vi "Write Setpoint Temperature.vi"(8 "error in (no error)":errorcluster, 9 "Update Time":timestamp, 10 "Setpoint Temperature [degC]":dbl, 11 "Thermal Chamber Response Simlator In":refnum<class "Thermal Chamber Response Simlator.lvclass">) -> (0 "error out":errorcluster, 3 "Thermal Chamber Response Simlator Out":refnum<class "Thermal Chamber Response Simlator.lvclass">)   [LabVIEW 2020, in "Thermal Chamber Response Simlator.lvclass"]
uses:
  Thermal Chamber Response Simlator.lvclass
  Thermal Chamber Response Simlator.lvclass/Thermal Chamber Response Simlator.ctl
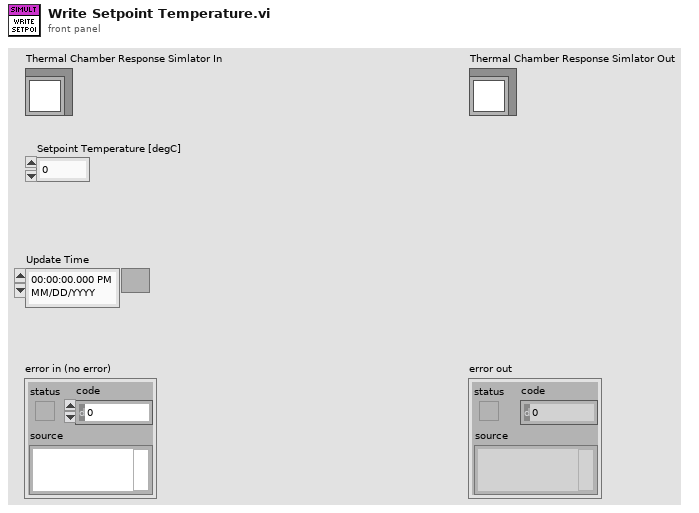
[diagram p1: front panel]
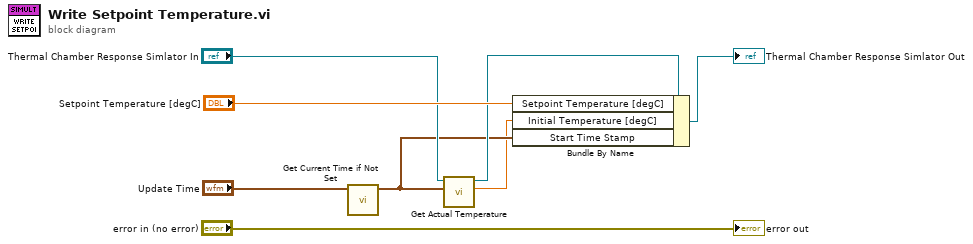
[diagram p0: block diagram]
diagram:
  n1 = call "Get Current Time if Not Set.vi"("Start Time"="Update Time") -> ("seconds since 1Jan1904"=w2:timestamp)  [unwired: 10 in]
  n2 = call "Get Actual Temperature.vi"("Time Stamp"=w2, "Thermal Chamber Response Simlator In"="Thermal Chamber Response Simlator In") -> ("Actual Temperature [degC]"=w1:dbl, "Thermal Chamber Response Simlator Out"=w3:refnum<class "Thermal Chamber Response Simlator.lvclass">)  [unwired: 7 in, 1 out]
  n3 = Bundle By Name(cluster=w3, "Setpoint Temperature [degC]"="Setpoint Temperature [degC]", "Initial Temperature [degC]"=w1, "Start Time Stamp"=w2) -> (→"Thermal Chamber Response Simlator Out":refnum<class "Thermal Chamber Response Simlator.lvclass">)
  "error out" <- "error in (no error)"
